vi "Autonomous Independent.vi"() -> ()   [LabVIEW 2020]
doc: "This VI is called when autonomous begins, and will automatically be terminated when autonomous ends. You can carry out timed or sensor driven robot movement independently without needing to return to the caller."
uses:
  Globals/FilePath_Globals.vi
panel:
  out "file text":string
  in  "play":string="TwoBallAuto.txt"
  out "Name of Play":string="FeedTest"
  out "DS Message":string
  out "Done":bool=TRUE
  # "Be sure to right-click and choose Data Operations>>Make Current Value default if you want to save the array values with the VI"
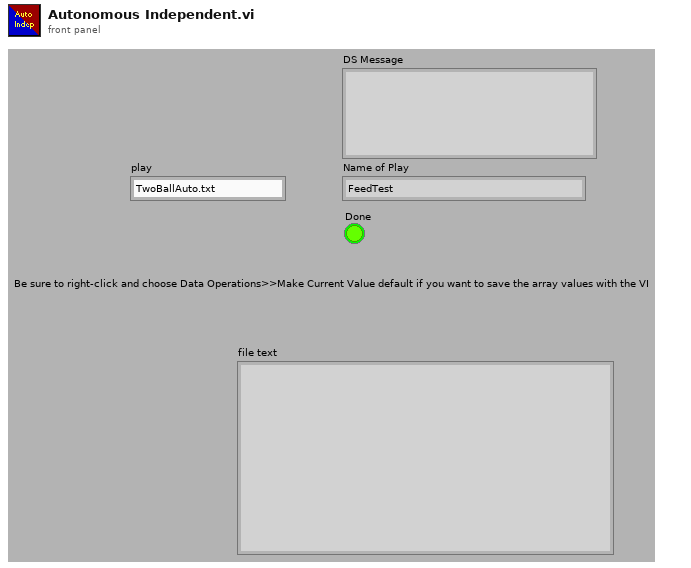
[diagram p1: front panel]
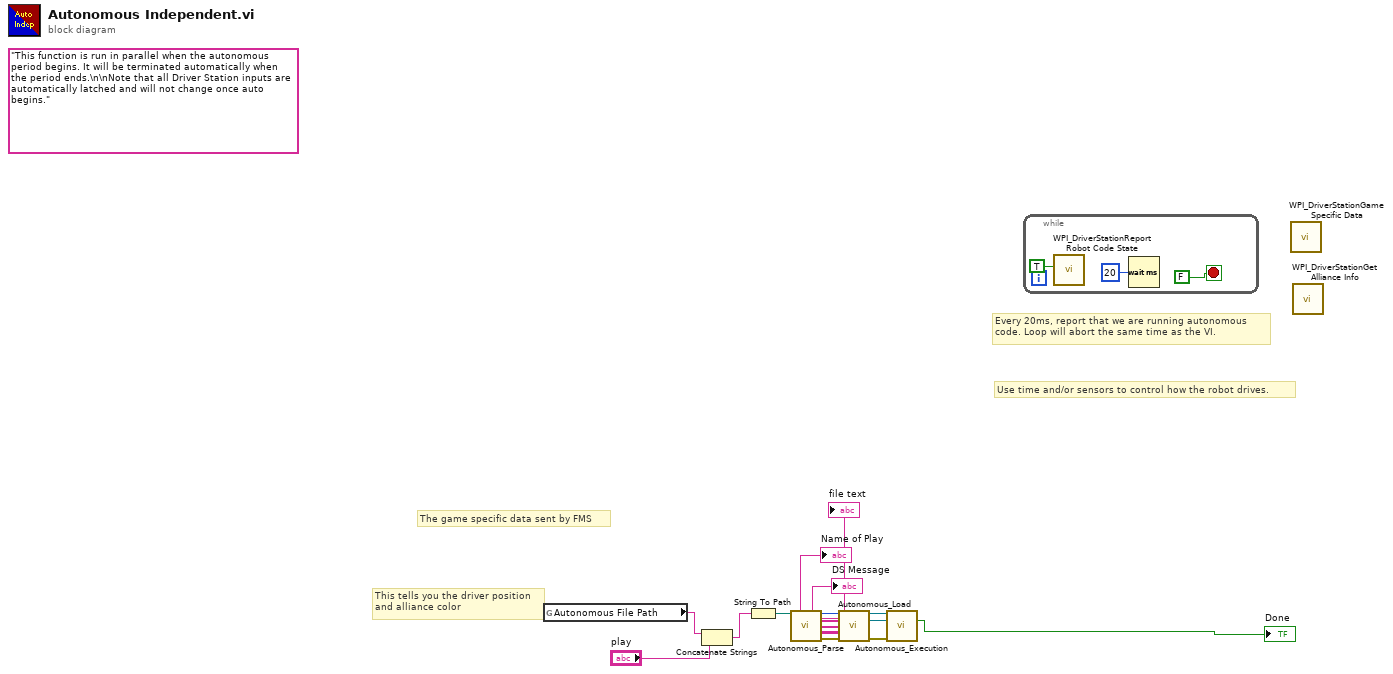
[diagram p0: block diagram]
diagram:
  (unwired) "This function is run in parallel when the autonomous period begins. It will be terminated automatically when the period ends.\n\nNote that all Driver Station inputs are automatically latched and will not change once auto begins."
  # "The game specific data sent by FMS"
  # "This tells you the driver position\nand alliance color"
  # "Every 20ms, report that we are running autonomous\ncode. Loop will abort the same time as the VI."
  # "Use time and/or sensors to control how the robot drives."
  n1 = global read "FilePath_Globals.vi" "Autonomous File Path"() -> (w4:string)
  n2 = Concatenate Strings(w4, "play") -> (w2:string)
  n3 = String To Path(string=w2) -> (path=w5:path)
  n4 = call "Autonomous_Parse.vi"("File Path"=w5) -> ("Name of Play"=→"Name of Play":string, "file text"=→"file text":string, "DS Message"=→"DS Message":string, "Number of Commands"=w15:i32, "Subsystems"=w14:string[], "Commands"=w13:string[], "Inputs"=w12:string[][], "errror out"=w11:errorcluster)  [unwired: 7 in]
  n5 = call "Autonomous_Load.vi"("Number of Commands"=w15, "Subsystems"=w14, "Commands"=w13, "Inputs"=w12, "error in"=w11) -> ("Queue_Key"=w8:refnum<queue>, "Autonomous_Queue"=w9:refnum<queue>, "errror out"=w10:errorcluster)  [unwired: 8 in]
  n6 = call "Autonomous_Execution.vi"("Queue Key"=w8, "Autonomous_Queue"=w9, "error in"=w10) -> ("Done"=→"Done":bool)  [unwired: 12 in]
  n7 = while {
    stop <- FALSE stop-if-true
    n8 = call <vilib>:"WPI_DriverStationReport Robot Code State.vi"("Autonomous"=TRUE) -> ()  [unwired: 10 in, 1 out]
    n9 = Wait (ms)(milliseconds to wait=u32 20) -> ()  [unwired: 1 out]
  }
  n10 = call <vilib>:"WPI_DriverStationGame Specific Data.vi"() -> ()  [unwired: 11 in, 1 out]
  n11 = call <vilib>:"WPI_DriverStationGet Alliance Info.vi"() -> ()  [unwired: 12 out]
